vi "AWS Execute CMD.vi"(8 "error in (no error)":errorcluster, 11 "LV-Data.AWS CLI":refnum<class "LV-Data.AWS CLI.lvclass">) -> (0 "error out":errorcluster, 2 "std out":string, 3 "LV-Data.AWS CLI out":refnum<class "LV-Data.AWS CLI.lvclass">)   [LabVIEW 2019, in "LV-Data.AWS CLI.lvclass"]
uses:
  LV-Data.AWS CLI.lvclass
panel:
  # "aws --version"
  # "aws s3 ls s3://levylab-data/CF900/"
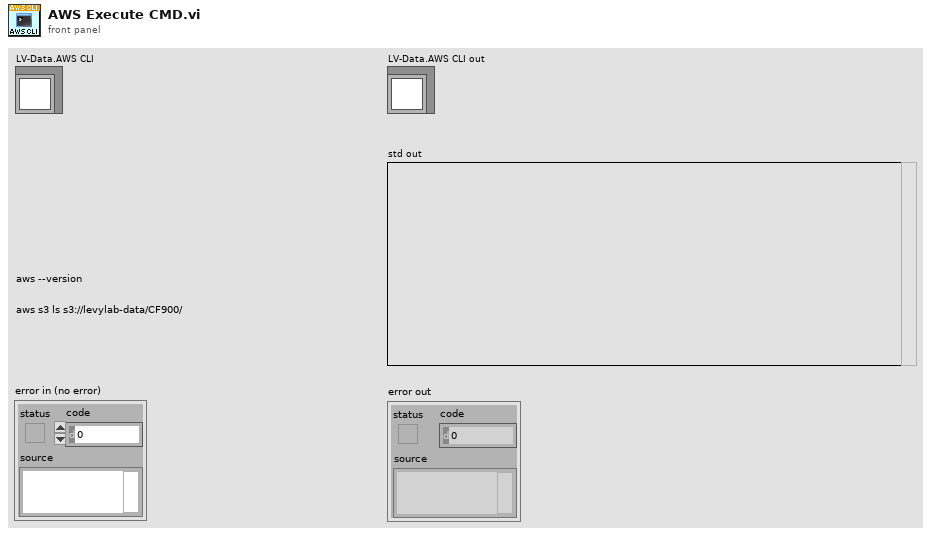
[diagram p1: front panel]
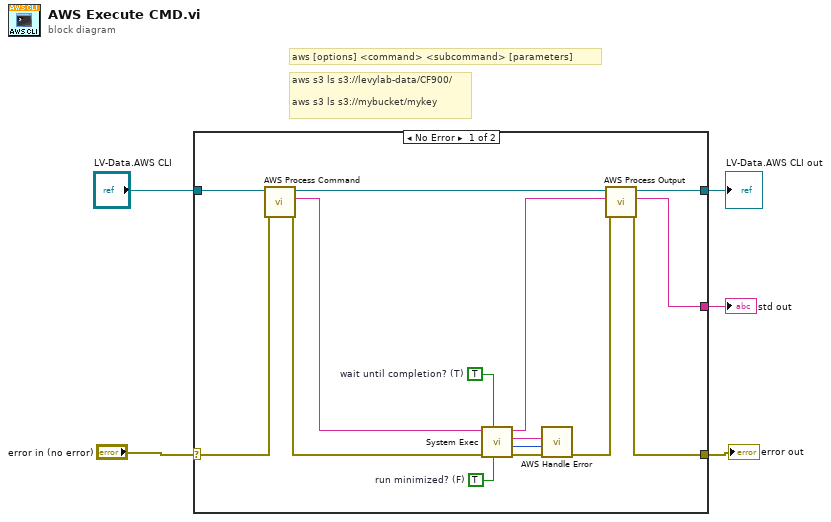
[diagram p0: block diagram]
diagram:
  # "aws s3 ls s3://levylab-data/CF900/\n\naws s3 ls s3://mybucket/mykey"
  # "aws [options] <command> <subcommand> [parameters]"
  n1 = case shown="No Error" "error in (no error)" {
    selector: "error in (no error)" -> [w15 w22]
    tunnel: [w11 w22] -> w4
    tunnel: [w9 w21] -> w2
    tunnel: "LV-Data.AWS CLI" -> [w6 w21]
    tunnel: [w8 _] -> w1
    frame No Error {
      w19 = TRUE  # wait until completion? (T)
      w20 = TRUE  # run minimized? (F)
      n2 = call "AWS Process Command.vi"("error in"=w15, "LV-Data.AWS CLI"=w6) -> ("error out"=w14:errorcluster, "command line"=w13:string, "LV-Data.AWS CLI out"=w10:refnum<class "LV-Data.AWS CLI.lvclass">)  [unwired: 7 in]
      n3 = call <vilib>:"System Exec.vi"("run minimized? (F)"=w20, "wait until completion? (T)"=w19, "error in (no error)"=w14, "command line"=w13) -> ("error out"=w18:errorcluster, "return code"=w16:i32, "standard error"=w17:string, "standard output"=w7:string)  [unwired: 4 in]
      n4 = call "AWS Handle Error.vi"("error in (no error)"=w18, "return code"=w16, "standard error"=w17) -> ("error out"=w12:errorcluster)  [unwired: 8 in]
      n5 = call "AWS Process Output.vi"("error in"=w12, "standard output"=w7, "LV-Data.AWS CLI"=w10) -> ("error out"=w11:errorcluster, "processed output"=w8:string, "LV-Data.AWS CLI out"=w9:refnum<class "LV-Data.AWS CLI.lvclass">)  [unwired: 6 in]
    }
    frame Error {
    }
  }
  "error out" <- w4
  "LV-Data.AWS CLI out" <- w2
  "std out" <- w1
